vi "US deaths data.vi"() -> ()   [LabVIEW 2019]
uses:
  <vilib>/httpClient/LabVIEWHTTPClient.lvlib
panel:
  out "populations":i32[](array[numeric])
  out "Deaths":i32[][](array[numeric])
  out "Array 3":string[](array[string])
  out "new deaths per day":i32[](array[numeric])
  out "days":i32[](array[numeric])
  in  "country index":u16
  out "cumulative deaths":i32[](array[numeric])
  out "first case date":timestamp
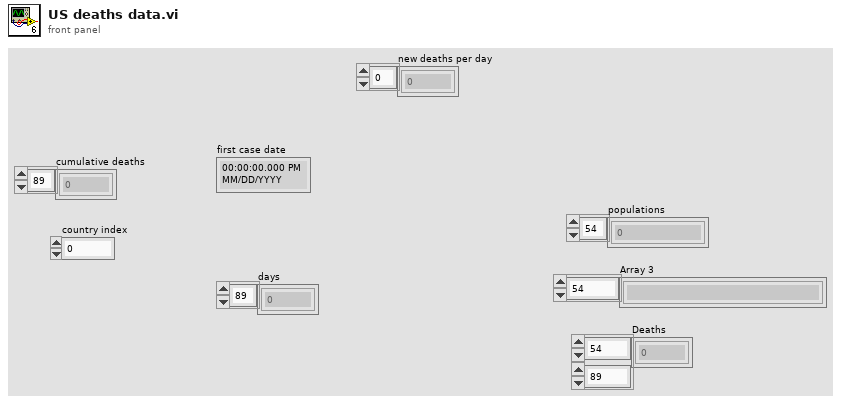
[diagram p1: front panel]
types:
  T1 = typedef "LabVIEWHTTPClient.lvlib/ClientHandle.ctl" = refnum<k1>
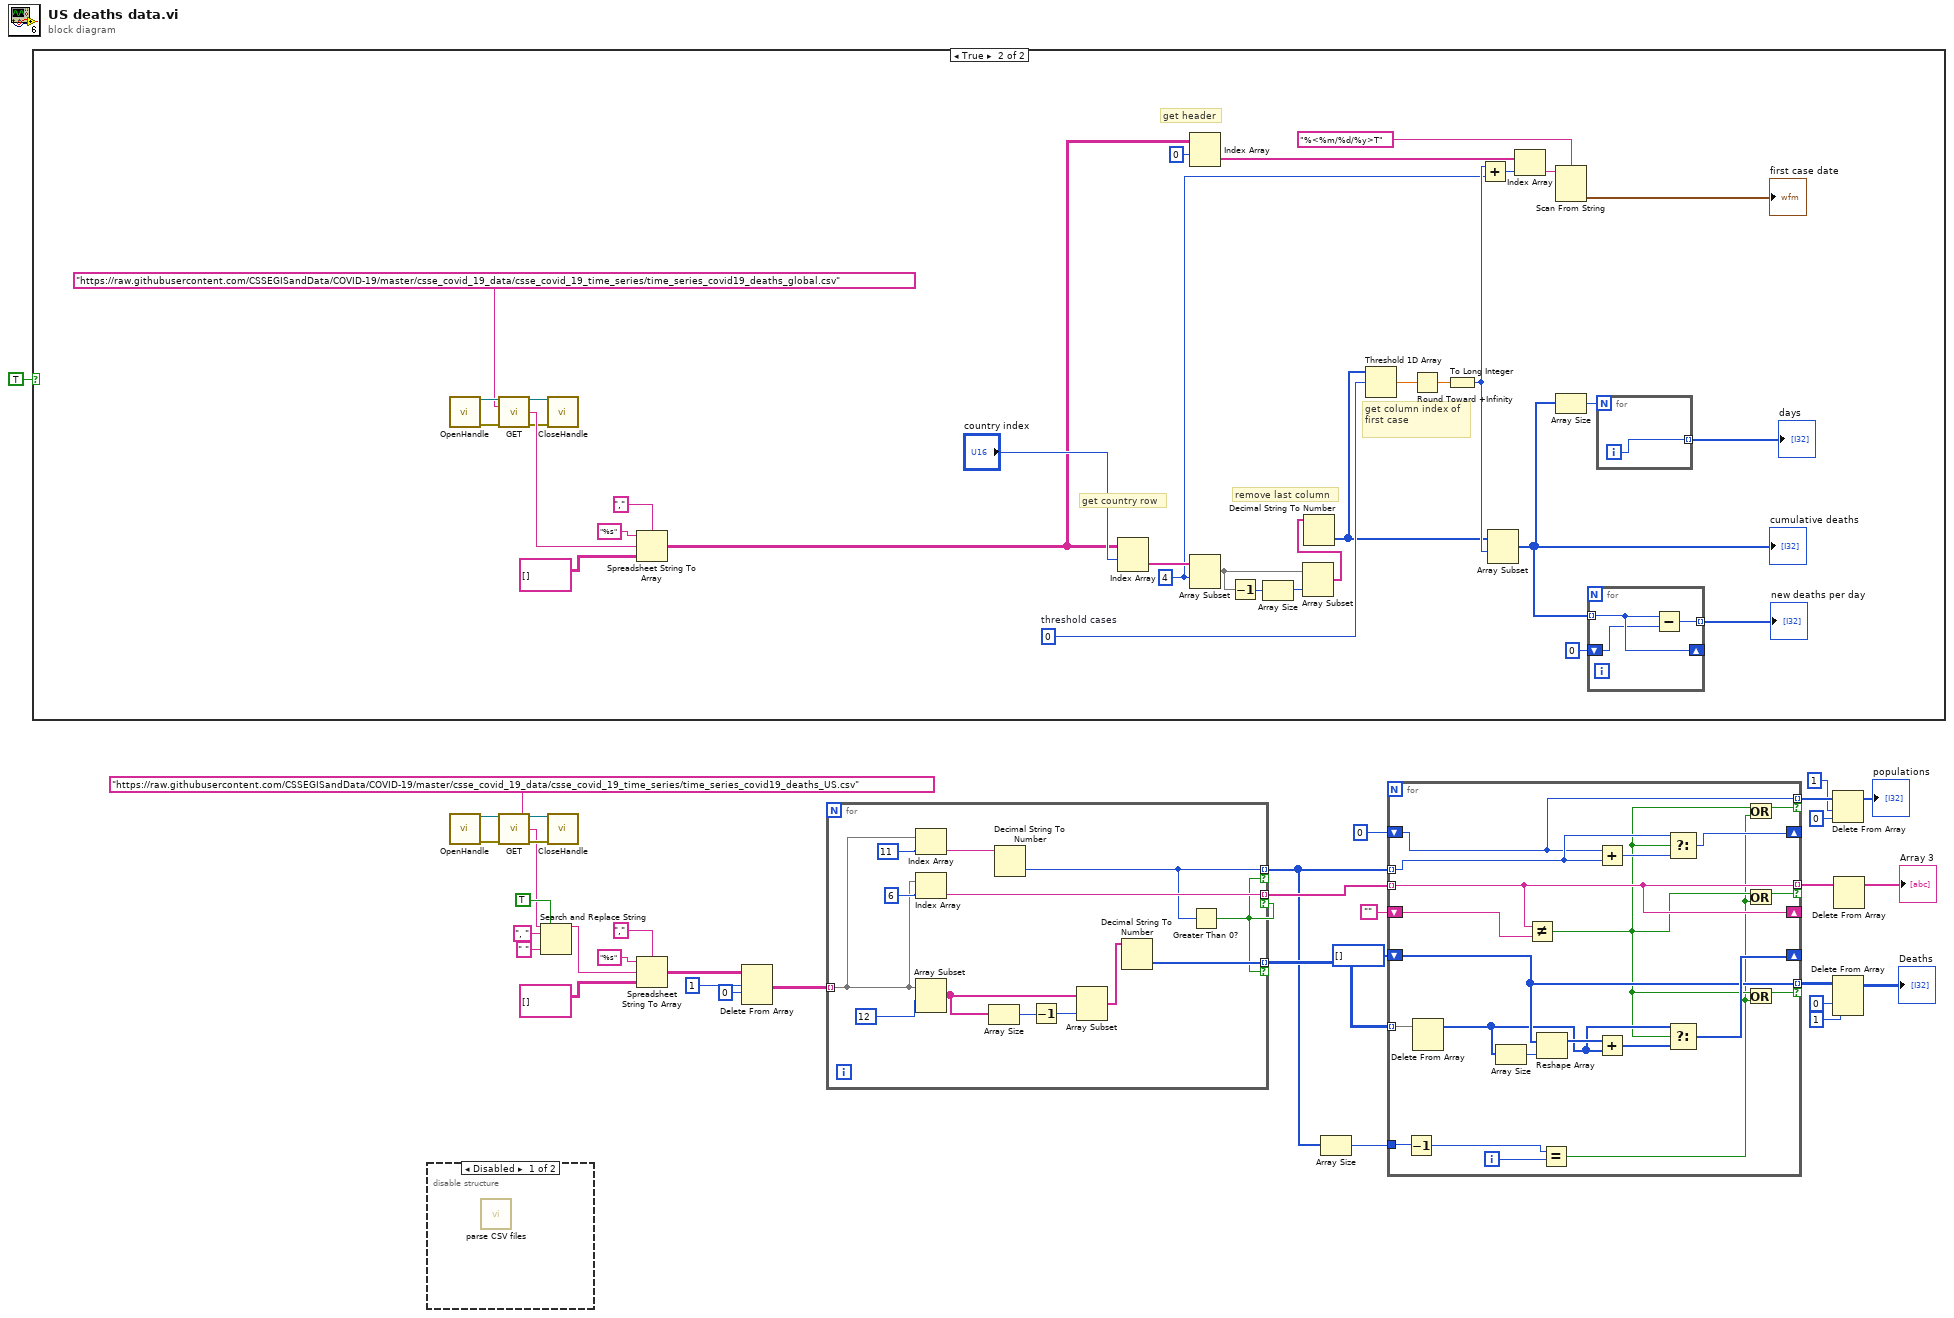
[diagram p0: block diagram]
diagram:
  n1 = case shown="True" TRUE {
    frame False {
    }
    frame True {
      w45 = u32 0  # threshold cases
      w37 = 4 ("index")
      # "get header"
      # "remove last column"
      # "get column index of first case"
      # "get country row"
      n2 = call <vilib>:"OpenHandle.vi"() -> ("client handle out"=w67:T1, "error out"=w66:errorcluster)  [unwired: 14 in]
      n3 = call <vilib>:"GET.vi"("client handle"=w67, "url"="https://raw.githubusercontent.com/CSSEGISandData/COVID-19/master/csse_covid_19_data/csse_covid_19_time_series/time_series_covid19_deaths_global.csv", "error in (no error)"=w66) -> ("client handle out"=w64:T1, "body"=w68:string, "error out"=w65:errorcluster)  [unwired: 9 in, 1 out]
      n4 = call <vilib>:"CloseHandle.vi"("client handle"=w64, "error in (no error)"=w65) -> ()  [unwired: 13 in, 1 out]
      n5 = Spreadsheet String To Array(delimiter (Tab)=",", format string="%s", spreadsheet string=w68, array type (2D Dbl)=string[][] []) -> (array=w36:string[][])
      n6 = Index Array(array=w36, index (row)="country index") -> (element=w47:string[])  [unwired: 1 in]
      n7 = Index Array(array=w36, index (row)=0) -> (element=w56:string[])  [unwired: 1 in]
      n8 = Array Subset(array=w47, index=w37) -> (w49:string[])  [unwired: 1 in]
      n9 = Array Size(array=w49) -> (size(s)=w50:i32)
      n10 = Decrement(x=w50) -> (x-1=w48:i32)
      n11 = Array Subset(array=w49, length=w48) -> (w51:string[])  [unwired: 1 in]
      n12 = Decimal String To Number(string=w51) -> (number=w38:i32[])  [unwired: 2 in, 1 out]
      n13 = Threshold 1D Array(2:w45, 3:w38) -> (0:w42:dbl)  [unwired: 1 in]
      n14 = Round Toward +Infinity(x=w42) -> (ceil(x): smallest int >= x=w43:dbl)
      n15 = To Long Integer(number=w43) -> (32bit integer=w58:i32)
      n16 = Add(x=w58, y=w37) -> (x+y=w54:i32)
      n17 = Array Subset(array=w38, index=w58) -> (w39:i32[])  [unwired: 1 in]
      "cumulative deaths" <- w39
      n18 = Index Array(array=w56, index=w54) -> (element=w53:string)
      n19 = Scan From String(format string="%<%m/%d/%y>T", input string=w53) -> (output 1=→"first case date":timestamp)  [unwired: 3 in, 3 out]
      n20 = Array Size(array=w39) -> (size(s)=w44:i32)
      n21 = for {
        tunnel: w39 -> [w71] mode=indexing
        shift-right: [w71] -> _
        shift-left: 0 -> [w70]
        tunnel: [w69] -> w40 mode=indexing
        n22 = Subtract(x=w71, y=w70) -> (x-y=w69:i32)
      }
      "new deaths per day" <- w40
      n23 = for {
        N: w44 -> [_]
        tunnel: [w72] -> w46 mode=indexing
        i -> [w72]
      }
      "days" <- w46
    }
  }
  n24 = disable-structure shown="Disabled" {
    frame Disabled {
      n25 = call "parse CSV files.vi"() -> ()  [unwired: 6 in, 6 out]
    }
    frame Enabled {
    }
  }
  n26 = call <vilib>:"OpenHandle.vi"() -> ("client handle out"=w28:T1, "error out"=w29:errorcluster)  [unwired: 14 in]
  n27 = call <vilib>:"GET.vi"("client handle"=w28, "url"="https://raw.githubusercontent.com/CSSEGISandData/COVID-19/master/csse_covid_19_data/csse_covid_19_time_series/time_series_covid19_deaths_US.csv", "error in (no error)"=w29) -> ("client handle out"=w31:T1, "body"=w20:string, "error out"=w30:errorcluster)  [unwired: 9 in, 1 out]
  n28 = Search and Replace String(replace all?=TRUE ("replace all? (F)"), input string=w20, search string=", ", replace string=" " ("replace string (\"\")")) -> (result string=w19:string)  [unwired: 4 in, 3 out]
  n29 = call <vilib>:"CloseHandle.vi"("client handle"=w31, "error in (no error)"=w30) -> ()  [unwired: 13 in, 1 out]
  n30 = Spreadsheet String To Array(delimiter (Tab)=",", format string="%s", spreadsheet string=w19, array type (2D Dbl)=string[][] []) -> (array=w26:string[][])
  n31 = Delete From Array(array=w26, length=1, index (row)=0) -> (array with subset deleted=w27:string[][])  [unwired: 1 in, 1 out]
  n32 = for {
    tunnel: w27 -> [w76] mode=indexing
    tunnel: [w79] -> w17 mode=indexing if=w73
    tunnel: [w78] -> w18 mode=indexing if=w73
    tunnel: [w74] -> w4 mode=indexing if=w73
    n33 = Index Array(array=w76, index=11) -> (element=w75:string)
    n34 = Index Array(array=w76, index=6) -> (element=w78:string)
    n35 = Array Subset(array=w76, index=12) -> (w84:string[])  [unwired: 1 in]
    n36 = Array Size(array=w84) -> (size(s)=w83:i32)
    n37 = Decimal String To Number(string=w75) -> (number=w74:i32)  [unwired: 2 in, 1 out]
    n38 = Decrement(x=w83) -> (x-1=w85:i32)
    n39 = Array Subset(array=w84, length=w85) -> (w82:string[])  [unwired: 1 in]
    n40 = Decimal String To Number(string=w82) -> (number=w79:i32[])  [unwired: 2 in, 1 out]
    n41 = Greater Than 0?(x=w74) -> (x > 0?=w73:bool)
  }
  n42 = Array Size(array=w4) -> (size(s)=w3:i32)
  n43 = for {
    tunnel: w18 -> [w105] mode=indexing
    tunnel: w17 -> [w99] mode=indexing
    shift-right: [w105] -> _
    shift-left: "" -> [w106]
    shift-right: [w104] -> _
    shift-left: i32[] [] -> [w100]
    tunnel: [w100] -> w14 mode=indexing if=w90
    tunnel: [w105] -> w1 mode=indexing if=w91
    tunnel: w4 -> [w96] mode=indexing
    shift-right: [w95] -> _
    shift-left: 0 -> [w94]
    tunnel: [w94] -> w8 mode=indexing if=w92
    tunnel: w3 -> [w88]
    i -> [w89]
    n44 = Decrement(x=w88) -> (x-1=w87:i32)
    n45 = Delete From Array(array=w99) -> (array with subset deleted=w98:i32[])  [unwired: 2 in, 1 out]
    n46 = Array Size(array=w98) -> (size(s)=w101:i32)
    n47 = Not Equal?(x=w105, y=w106) -> (x != y?=w93:bool)
    n48 = Reshape Array(w100, w101) -> (w102:i32[])
    n49 = Equal?(x=w87, y=w89) -> (x = y?=w86:bool)
    n50 = Add(x=w94, y=w96) -> (x+y=w97:i32)
    n51 = Add(x=w102, y=w98) -> (x+y=w103:i32[])
    n52 = Select(t=w96, s=w93, f=w97) -> (s? t:f=w95:i32)
    n53 = Select(t=w98, s=w93, f=w103) -> (s? t:f=w104:i32[])
    n54 = Or(x=w93, y=w86) -> (x .or. y?=w92:bool)
    n55 = Or(x=w93, y=w86) -> (x .or. y?=w91:bool)
    n56 = Or(x=w93, y=w86) -> (x .or. y?=w90:bool)
  }
  n57 = Delete From Array(array=w8, length=1, index=0 ("index (row)")) -> (array with subset deleted=→"populations":i32[])  [unwired: 1 out]
  n58 = Delete From Array(array=w14, length=1, index (row)=0) -> (array with subset deleted=→"Deaths":i32[][])  [unwired: 1 in, 1 out]
  n59 = Delete From Array(array=w1) -> (array with subset deleted=→"Array 3":string[])  [unwired: 2 in, 1 out]
